vi "Task Killer.vi"   [LabVIEW 2014, in "Managing Executables.lvlib"]
uses:
  Managing Executables.lvlib
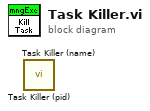
[diagram p0: block diagram]
diagram:
  n1 = call "Task Killer (pid).vi"() -> ()  [unwired: 7 in, 1 out]
  n2 = call "Task Killer (name).vi"() -> ()  [unwired: 7 in, 1 out]
